vi "SliderDual.vi"() -> ()   [LabVIEW 2020]
panel:
  in  "Value":dbl
  out "Display":cluster{dbl, dbl}(slide)={0.0, 5.948553054662379} scale=-10.0..10.0
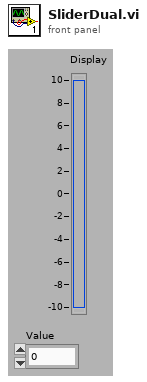
[diagram p1: front panel]
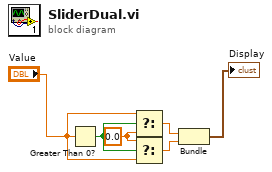
[diagram p0: block diagram]
diagram:
  w5 = 0.0 ("f")
  n1 = Greater Than 0?(x="Value") -> (x > 0?=w6:bool)
  n2 = Select(t="Value", s=w6, f=w5) -> (s? t:f=w3:dbl)
  n3 = Select(t=w5, s=w6, f="Value") -> (s? t:f=w2:dbl)
  n4 = Bundle("f"=w3, "Value"=w2) -> (→"Display":cluster{"f":dbl, "Value":dbl})  [unwired: 1 in]
